vi "any tabs open.vi"() -> (3 "any tabs open?":bool)   [LabVIEW 2012]
uses:
  GFG/GFGbooleanGet.vi
  GFG/GFG library.lvlib
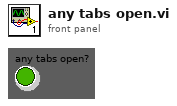
[diagram p1: front panel]
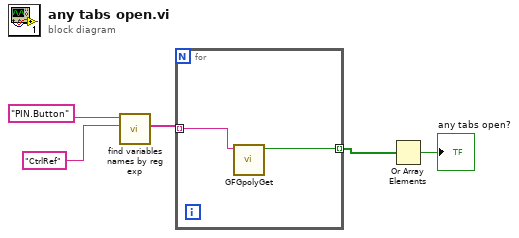
[diagram p0: block diagram]
diagram:
  n1 = call "find variables  names by reg exp.vi"("exclude string (reg exp)"="CtrlRef", "search string (reg exp)"="PIN.Button" ("exclude string (reg exp)")) -> ("Array of Variable Names"=w1:string[])  [unwired: 8 in, 1 out]
  n2 = for {
    tunnel: w1 -> [w7] mode=indexing
    tunnel: [w6] -> w5 mode=indexing
    n3 = call-poly "GFGpolyGet.vi"("Variable Name in"=w7) -> ("Boolean"=w6:bool)  [unwired: 10 in]
  }
  n4 = Or Array Elements(Boolean array=w5) -> (logical OR=→"any tabs open?":bool)
